vi "Library - Child Libraries.vi"(7 "Msg Chain":string, 8 "error in (no error)":errorcluster {"code" format="Error %.0f"}, 10 "Libraries":refnum<class "Library Documentation.lvclass">[](array[class]), 11 "VIDoc Printer - Confluence In":refnum<class "VIDoc Printer - Confluence.lvclass">) -> (0 "error out":errorcluster {"code" format="Error %.0f"}, 3 "VIDoc Printer - Confluence Out":refnum<class "VIDoc Printer - Confluence.lvclass">)   [LabVIEW 2023, in "VIDoc Printer - Confluence.lvlib" / "VIDoc Printer - Confluence.lvclass"]
uses:
  VIDoc Printer - Confluence.lvclass
  C:/projects/DMC/GitHub/DMC CLI VIDoc/Source/Documentation Generation/Printers/Printer/VIDoc Printer.lvclass
  Parsing/Library Documentation/Library Documentation.lvclass
  Printer/VIDoc Printer.lvclass/VIDoc Printer.ctl
  Parsing/Library Documentation/Library Documentation.lvclass/Library Documentation.ctl
  Confluence Formatting/Types/Format Combo Box.ctl
  VIDoc Printer - Confluence.lvclass/VIDoc Printer - Confluence.ctl
  Accessors/Get Library Inheritance Expand.vi
  Printer/Accessors/Get Library Scope.vi
  Parsing/Library Documentation/Get Child Libraries.vi
  Parsing/Library Documentation/Get Name.vi
  Printer/VIDoc Printer.lvclass
  UI Interaction/UI Interaction.lvclass
  Confluence Formatting/Confluence Formatting.lvlib
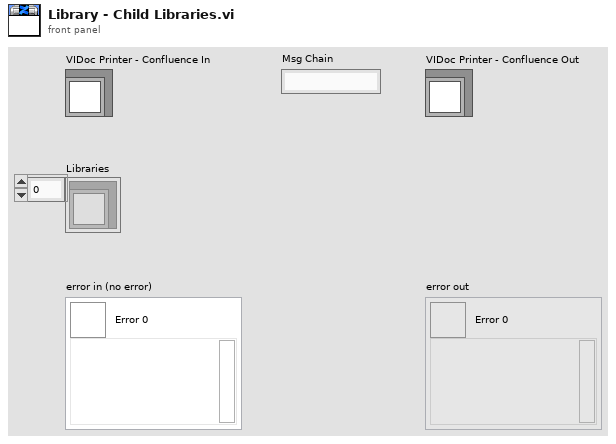
[diagram p1: front panel]
types:
  T1 = typedef "Confluence Formatting.lvlib/Format Combo Box.ctl" = string
  T2 = typedef "VIDoc Parsing.lvlib/Library Documentation.lvclass/Child Libraries Cluster.ctl" = cluster{"Qualified Name":string, "Library Scope":enum32{"invalid scope", "public", "private", "protected", "community"}}
  T3 = cluster{"Public":bool, "Community":bool, "Private":bool, "Unknown":bool}
  T4 = enum32{"invalid scope", "public", "private", "protected", "community"}
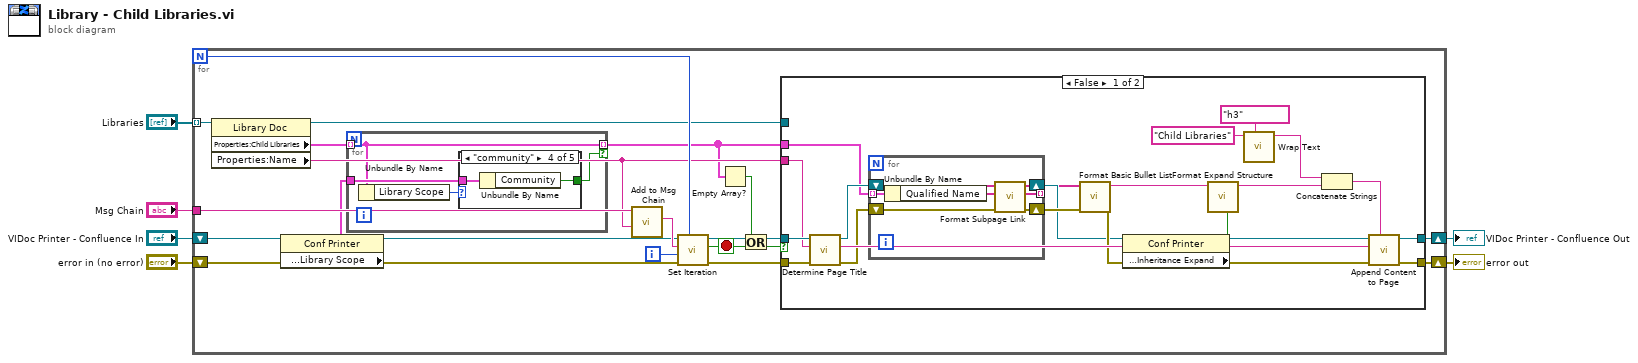
[diagram p0: block diagram]
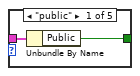
[diagram p2: hidden frame]
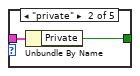
[diagram p3: hidden frame]
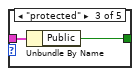
[diagram p4: hidden frame]
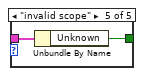
[diagram p5: hidden frame]
diagram:
  n1 = for {
    N -> [w19]
    shift-right: [w24] -> w2
    shift-left: "error in (no error)" -> [w22]
    shift-right: [w25] -> w1
    shift-left: "VIDoc Printer - Confluence In" -> [w23]
    tunnel: "Libraries" -> [w26] mode=indexing
    tunnel: "Msg Chain" -> [w17]
    i -> [w18]
    stop <- w14 stop-if-true
    n2 = property class="Library Doc"(reference=w26) -> (reference out=w13:refnum<class "Library Documentation.lvclass">, "Properties:Child Libraries"=w9:T2[], "Properties:Name"=w16:string)  [unwired: 1 in, 1 out]
    n3 = property class="Conf Printer"(reference=w23) -> (reference out=w10:refnum<class "VIDoc Printer - Confluence.lvclass">, "Properties:Settings:Library Scope:Library Scope"=w8:T3)  [unwired: 1 in, 1 out]
    n4 = for {
      tunnel: w8 -> [w29]
      tunnel: [w27] -> w7 mode=indexing if=w28
      tunnel: w9 -> [w27] mode=indexing
      n5 = Unbundle By Name(w27) -> ("Library Scope"=w30:T4)
      n6 = case shown="\"community\"" w30 {
        tunnel: w29 -> [w32 w34 w36 w38 w40]
        tunnel: [w31 w33 w35 w37 w39] -> w28
        frame "public" {
          n7 = Unbundle By Name(w32) -> ("Public"=w31:bool)
        }
        frame "private" {
          n8 = Unbundle By Name(w34) -> ("Private"=w33:bool)
        }
        frame "protected" {
          n9 = Unbundle By Name(w36) -> ("Public"=w35:bool)
        }
        frame "community" {
          n10 = Unbundle By Name(w38) -> ("Community"=w37:bool)
        }
        frame "invalid scope" {
          n11 = Unbundle By Name(w40) -> ("Unknown"=w39:bool)
        }
      }
    }
    n12 = call "Add to Msg Chain.vi"("New"=w16, "Msg Chain in"=w17) -> ("Msg Chain out"=w15:string)  [unwired: 9 in]
    n13 = call "Set Iteration.vi"("Progress Max"=w19, "error in (no error)"=w22, "Progress Value"=w18, "Message (No Message Update)"=w15, "VIDoc Printer In"=w10) -> ("error out"=w20:errorcluster, "Abort?"=w14:bool, "VIDoc Printer Out"=w21:refnum<class "VIDoc Printer - Confluence.lvclass">)  [unwired: 4 in]
    n14 = Empty Array?(array=w7) -> (empty?=w11:bool)
    n15 = Or(x=w11, y=w14) -> (x .or. y?=w12:bool)
    n16 = case shown="False" w12 {
      tunnel: [w60 w69] -> w25
      tunnel: [w59 w70] -> w24
      tunnel: w21 -> [w57 w69]
      tunnel: w20 -> [w56 w70]
      tunnel: w16 -> [w55 _]
      tunnel: w13 -> [_ _]
      tunnel: w7 -> [w41 _]
      frame False {
        n17 = call "Determine Page Title.vi"("error in (no error)"=w56, "Name"=w55, "VIDoc Printer - Confluence In"=w57) -> ("error out"=w46:errorcluster, "Page Title"=w61:string, "VIDoc Printer - Confluence Out"=w44:refnum<class "VIDoc Printer - Confluence.lvclass">)  [unwired: 5 in, 1 out]
        n18 = for {
          shift-right: [w67] -> w45
          shift-left: w46 -> [w68]
          shift-right: [w65] -> w43
          shift-left: w44 -> [w66]
          tunnel: w41 -> [w64] mode=indexing
          tunnel: [w63] -> w42 mode=indexing
          n19 = Unbundle By Name(w64) -> ("Qualified Name"=w62:string)
          n20 = call "Format Subpage Link.vi"("error in (no error)"=w68, "Qualified Name"=w62, "VIDoc Printer - Confluence In"=w66) -> ("error out"=w67:errorcluster, "Linked HTML"=w63:string, "VIDoc Printer - Confluence Out"=w65:refnum<class "VIDoc Printer - Confluence.lvclass">)  [unwired: 6 in]
        }
        n21 = call "Format Basic Bullet List.vi"("Error in"=w45, "String Array"=w42) -> ("Error out"=w51:errorcluster, "Bullet List"=w50:string)  [unwired: 8 in]
        n22 = property class="Conf Printer"(reference=w43) -> (reference out=w49:refnum<class "VIDoc Printer - Confluence.lvclass">, "Properties:Expand?:Library:Inheritance Expand"=w47:bool)  [unwired: 1 in, 1 out]
        n23 = call "Format Expand Structure.vi"("Enable? (T)"=w47, "Content"=w50) -> ("Expand String"=w48:string)  [unwired: 8 in, 1 out]
        n24 = call "Wrap Text.vi"("Formatting"=T1 "h3", "String"="Child Libraries") -> ("Wrapped String"=w53:string)  [unwired: 8 in, 1 out]
        n25 = Concatenate Strings(w53, w48) -> (w52:string)
        n26 = call "Append Content to Page.vi"("Page Content"=w52, "error in (no error)"=w51, "Page Title"=w61, "VIDoc Printer - Confluence In"=w49) -> ("error out"=w59:errorcluster, "VIDoc Printer - Confluence Out"=w60:refnum<class "VIDoc Printer - Confluence.lvclass">)  [unwired: 6 in]
      }
      frame True {
      }
    }
  }
  "error out" <- w2
  "VIDoc Printer - Confluence Out" <- w1
